vi "lvEtherbone.device_open.vi"(0 "eb_socket_ID":i32, 1 "ip_port":string, 2 "proposed_widths":T1=15 items=["EB_DATA8"=1, "EB_DATA16"=2, "EB_DATA32"=4, "EB_DATA64"=8, "EB_DATAX"=15], 5 "error in (no error)":errorcluster) -> (13 "eb_status":T2, 14 "eb_socket_ID out":i32, 15 "eb_device_ID":i32, 19 "error out":errorcluster)   [LabVIEW 2009, in "lvEtherbone.lvlib"]
doc: "//-----------------------------------------------------------------------------------\n// author : Dietrich Beck, GSI-Darmstadt\n// purpose : Open a remote Etherbone device.\n// This resolves the address and performs Etherbone end-point discovery.\n// From the mask of proposed bus widths, one will be selected.\n// The default port is taken as 0xEBD0.Detach the device from the virtual bus.\n// returns : lveb_status_t\n//-----------------------------------------------------------------------------------\nETHERBONE_API int lveb_device_open( int eb_socketID, //Etherbone socket ID\n char *ip_port, //IP port in the format \"IP:PORT\"\n int proposed_widths, //width of Wishbone bus\n int *eb_deviceID //Wishbone device ID\n );"
uses:
  lvEtherbone.lvlib
  lvEtherbone.lveb_status_t.ctl
  lvEtherbone.eb_width_t.ctl
  bin/lvEtherbone.dll
panel:
  in  "eb_status_t":T2
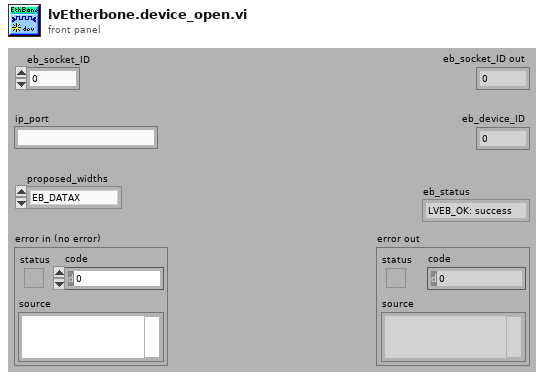
[diagram p1: front panel]
types:
  T1 = typedef "lvEtherbone.lvlib/lvEtherbone.eb_width_t.ctl" = u32
  T2 = typedef "lvEtherbone.lvlib/lvEtherbone.lveb_status_t.ctl" = enum32{"LVEB_OK: success", "LVEB_UNKNOWN: unknown error", "LVEB_OS: operating system forbids access", "LVEB_PORT: port in use or unavailable", "LVEB_ID: ID invalid or out of resources", "LVEB_SOCKET: socket invalid or unavailable", "LVEB_EB: remote address is not Etherbone conformant", "LVEB_IP: bad format or network address", "LVEB_BUSWIDTH: bus width error", "LVEB_DEVICEBUSY: Whishbone device still busy", "LVEB_DEVICEFAIL: operation on Wishbone device failed", "LVEB_DEVICEEXIST: Whishbone device already exists, overlaps, or does not exist", "LVEB_TIMEDOUT: a timeout occurred", "LVEB_OVERFLOW: payload of Etherbone exceeded", "LVEB_ADDRESS: bad address"}
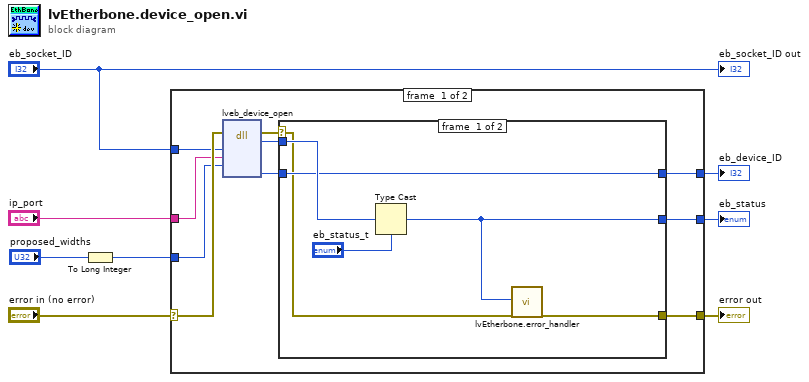
[diagram p0: block diagram]
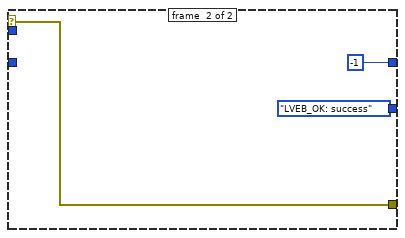
[diagram p2: hidden frame]
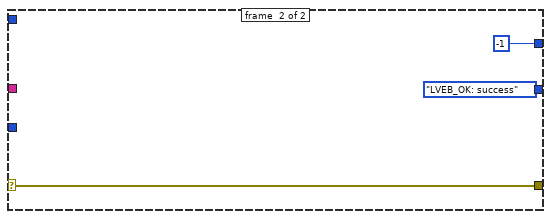
[diagram p3: hidden frame]
diagram:
  n1 = To Long Integer(number="proposed_widths") -> (32bit integer=w1:i32)
  n2 = case shown="No Error" "error in (no error)" {
    selector: "error in (no error)" -> [w18 w30]
    tunnel: [w15 w30] -> w7
    tunnel: "eb_socket_ID" -> [w9 _]
    tunnel: "ip_port" -> [w12 _]
    tunnel: [w16 lvEtherbone.lveb_status_t."LVEB_OK: success" ("eb_status_t")] -> w5
    tunnel: [w14 -1 ("eb_socket_ID")] -> w4
    tunnel: w1 -> [w11 _]
    frame #0 {
      n3 = dll-call lib="F:/beck/Project/BEL/SCC/etherbone-core/api/lvEtherbone/bin/lvEtherbone.*" fn="lveb_device_open"(error in=w18, "eb_socket_ID"=w9, "ip_port"=w12, "proposed_widths"=w11) -> (error out=w13:errorcluster, "eb_status"=w17:i32, "eb_device_ID"=w10:i32)  [unwired: 6 in, 1 out]
      n4 = case shown="No Error" w13 {
        selector: w13 -> [w19 w27]
        tunnel: w17 -> [w24 _]
        tunnel: [w21 lvEtherbone.lveb_status_t."LVEB_OK: success" ("eb_status_t")] -> w16
        tunnel: [w20 w27] -> w15
        tunnel: w10 -> [w23 _]
        tunnel: [w23 -1 ("eb_socket_ID")] -> w14
        frame #0 {
          n5 = Type Cast(type="eb_status_t", x=w24) -> (*(type *) &x=w21:T2)
          n6 = call "lvEtherbone.error_handler.vi"("eb_status"=w21, "error in"=w19) -> ("error out"=w20:errorcluster)  [unwired: 17 in]
        }
        frame #1 {
        }
      }
    }
    frame #1 {
    }
  }
  "error out" <- w7
  "eb_status" <- w5
  "eb_device_ID" <- w4
  "eb_socket_ID out" <- "eb_socket_ID"
